vi "Phasor Apply-Cancel Calibration.vi"(4 "Apply(T)/Cancel Calibration":bool=TRUE, 6 "Calibrated Phasor":bool, 8 "Error In":errorcluster, 9 "Target Phasor":cxt, 10 "Calibration Phasor":cxt, 11 "Phasor in":cxt) -> (0 "Error Out":errorcluster, 3 "Phasor out":cxt)   [LabVIEW 2021, in "Phasor.lvlib"]
doc: "<B>Phasor in</B> = z_in\n\n<B>Calibration Phasor</B> = z_c\n\n<B>Target Phasor</B> = z_t\n\n<B>Phasor out</B> = z_out\n\nApply Calibration: z_out = z_in*z_t/z_c\n\nCancel Calibration: z_out = z_in*z_c/z_t"
uses:
  Phasor.lvlib
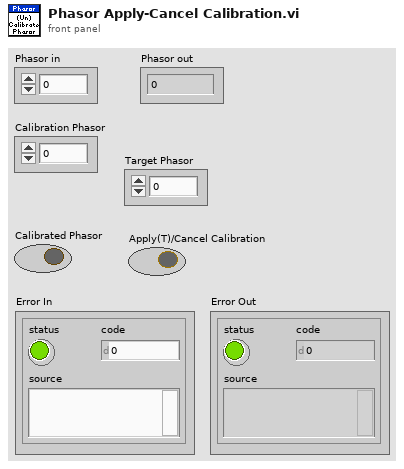
[diagram p1: front panel]
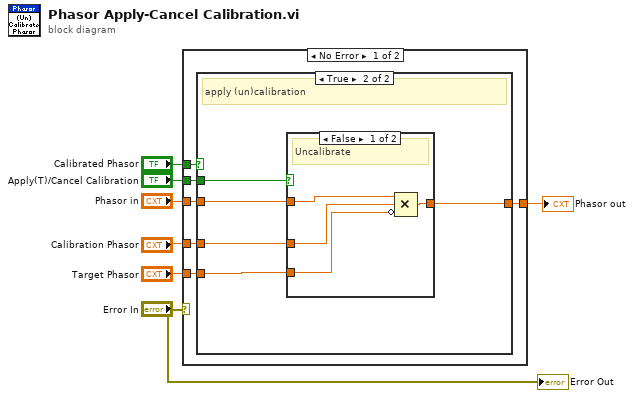
[diagram p0: block diagram]
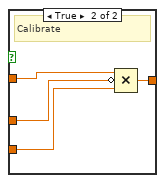
[diagram p3: hidden frame]
diagram:
  n1 = case shown="No Error" "Error In" {
    tunnel: "Calibration Phasor" -> [w13 _]
    tunnel: "Phasor in" -> [w12 w28]
    tunnel: [w11 w28] -> w5
    tunnel: "Calibrated Phasor" -> [w10 _]
    tunnel: "Target Phasor" -> [w9 _]
    tunnel: "Apply(T)/Cancel Calibration" -> [w8 _]
    frame No Error {
      n2 = case shown="True" w10 {
        tunnel: w13 -> [_ w19]
        tunnel: w12 -> [w14 w18]
        tunnel: [w14 w17] -> w11
        tunnel: w9 -> [_ w16]
        tunnel: w8 -> [_ w15]
        frame False {
          # "Ignore (un)calibration"
        }
        frame True {
          # "apply (un)calibration"
          n3 = case shown="False" w15 {
            tunnel: w18 -> [w23 w27]
            tunnel: w19 -> [w22 w26]
            tunnel: w16 -> [w21 w25]
            tunnel: [w20 w24] -> w17
            frame False {
              # "Uncalibrate"
              n4 = Compound Arithmetic op=MULTIPLY(w23, w22, invert w21) -> (w20:cxt)
            }
            frame True {
              # "Calibrate"
              n5 = Compound Arithmetic op=MULTIPLY(w27, invert w26, w25) -> (w24:cxt)
            }
          }
        }
      }
    }
    frame Error {
    }
  }
  "Phasor out" <- w5
  "Error Out" <- "Error In"
